vi "对称性1.vi"(11 "XY图":cluster{dbl[], dbl[]}[](graph)) -> (3 "对称性":dbl)   [LabVIEW 2019]
uses:
  <vilib>/Analysis/NI_AAL_Geometry.lvlib
panel:
  out "右":dbl
  out "左":dbl
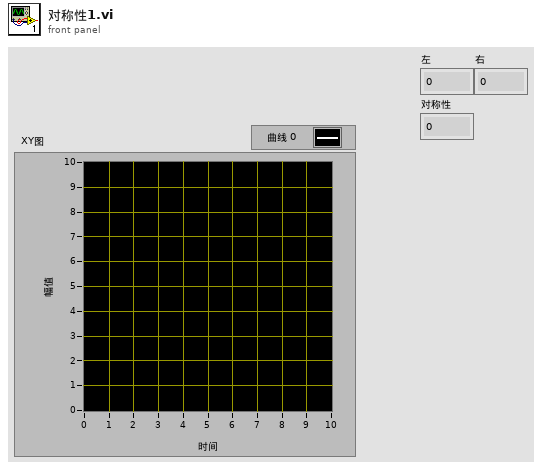
[diagram p1: front panel]
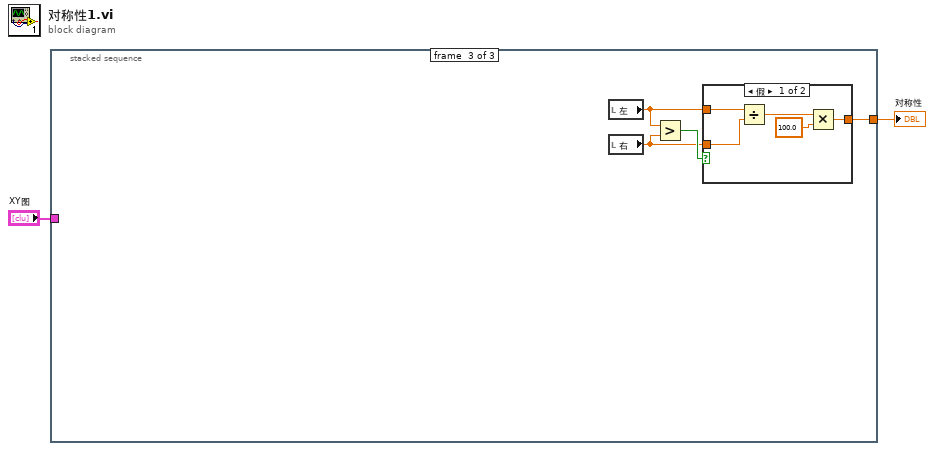
[diagram p0: block diagram]
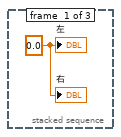
[diagram p2: hidden frame]
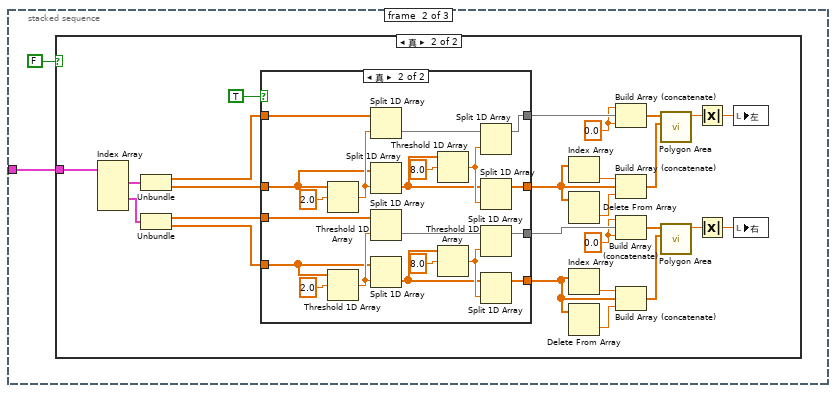
[diagram p3: hidden frame]
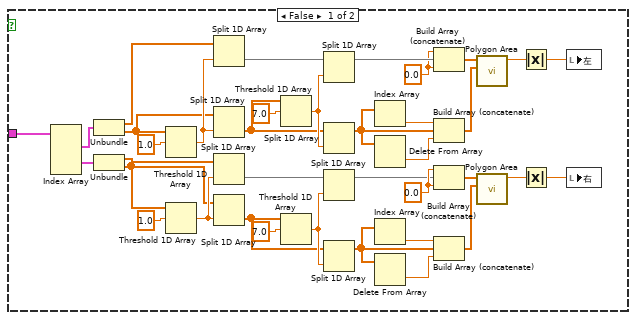
[diagram p4: hidden frame]
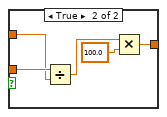
[diagram p6: hidden frame]
diagram:
  n1 = stacked-sequence {
    tunnel: "XY图" -> [_ w4 _]
    tunnel: [_ _ w93] -> w2
    frame #0 {
      w3 = 0.0 ("左")
      "左" <- w3
      "右" <- w3
    }
    frame #1 {
      n2 = case shown="真" FALSE {
        tunnel: w4 -> [w36 w44]
        frame False {
          w10 = 0.0
          w18 = 0.0
          n3 = Index Array(array=w36) -> (element #1=w37:cluster{dbl[], dbl[]}, element #3=w38:cluster{dbl[], dbl[]})  [unwired: 4 in, 2 out]
          n4 = Unbundle(w37) -> (w34:dbl[], w28:dbl[])
          n5 = Unbundle(w38) -> (w29:dbl[], w30:dbl[])
          n6 = Threshold 1D Array(2:1.0 ("阈值y"), 3:w28) -> (0:w33:dbl)  [unwired: 1 in]
          n7 = Threshold 1D Array(2:1.0 ("阈值y"), 3:w30) -> (0:w32:dbl)  [unwired: 1 in]
          n8 = Split 1D Array(array=w34, index=w33) -> (second subarray=w25:dbl[])  [unwired: 1 out]
          n9 = Split 1D Array(array=w28, index=w33) -> (second subarray=w24:dbl[])  [unwired: 1 out]
          n10 = Split 1D Array(array=w29, index=w32) -> (second subarray=w21:dbl[])  [unwired: 1 out]
          n11 = Split 1D Array(array=w30, index=w32) -> (second subarray=w20:dbl[])  [unwired: 1 out]
          n12 = Threshold 1D Array(2:7.0 ("阈值y"), 3:w24) -> (0:w27:dbl)  [unwired: 1 in]
          n13 = Threshold 1D Array(2:7.0 ("阈值y"), 3:w20) -> (0:w22:dbl)  [unwired: 1 in]
          n14 = Split 1D Array(array=w25, index=w27) -> (first subarray=w19:dbl[])  [unwired: 1 out]
          n15 = Split 1D Array(array=w24, index=w27) -> (first subarray=w16:dbl[])  [unwired: 1 out]
          n16 = Split 1D Array(array=w21, index=w22) -> (first subarray=w8:dbl[])  [unwired: 1 out]
          n17 = Split 1D Array(array=w20, index=w22) -> (first subarray=w9:dbl[])  [unwired: 1 out]
          n18 = Index Array(array=w16) -> (element=w17:dbl)  [unwired: 1 in]
          n19 = Delete From Array(array=w16) -> (deleted portion=w15:dbl)  [unwired: 2 in, 1 out]
          n20 = Index Array(array=w9) -> (element=w11:dbl)  [unwired: 1 in]
          n21 = Delete From Array(array=w9) -> (deleted portion=w12:dbl)  [unwired: 2 in, 1 out]
          n22 = Build Array (concatenate)(w18, w19, w18) -> (w14:dbl[])
          n23 = Build Array (concatenate)(w17, w16, w15) -> (w13:dbl[])
          n24 = Build Array (concatenate)(w10, w8, w10) -> (w7:dbl[])
          n25 = Build Array (concatenate)(w11, w9, w12) -> (w6:dbl[])
          n26 = call <vilib>:"Polygon Area.vi"("Y"=w13, "X"=w14) -> ("signed area"=w39:dbl)  [unwired: 8 in, 1 out]
          n27 = call <vilib>:"Polygon Area.vi"("Y"=w6, "X"=w7) -> ("signed area"=w41:dbl)  [unwired: 8 in, 1 out]
          n28 = Absolute Value(x=w39) -> (abs(x)=w40:dbl)
          n29 = Absolute Value(x=w41) -> (abs(x)=w42:dbl)
          n30 = local write "左"(w40) -> ()
          n31 = local write "右"(w42) -> ()
        }
        frame True {
          w46 = 0.0
          w45 = 0.0
          n32 = Index Array(array=w44) -> (element #1=w63:cluster{dbl[], dbl[]}, element #3=w64:cluster{dbl[], dbl[]})  [unwired: 4 in, 2 out]
          n33 = Unbundle(w63) -> (w62:dbl[], w59:dbl[])
          n34 = Unbundle(w64) -> (w60:dbl[], w61:dbl[])
          n35 = case shown="真" TRUE {
            tunnel: w62 -> [w72 w92]
            tunnel: w61 -> [w69 w89]
            tunnel: w60 -> [w70 w88]
            tunnel: w59 -> [w71 w87]
            tunnel: [w72 w80] -> w58
            tunnel: [w71 w79] -> w56
            tunnel: [w69 w78] -> w50
            tunnel: [w70 w77] -> w49
            frame False {
            }
            frame True {
              n36 = Threshold 1D Array(2:2.0 ("阈值y"), 3:w87) -> (0:w91:dbl)  [unwired: 1 in]
              n37 = Threshold 1D Array(2:2.0 ("阈值y"), 3:w89) -> (0:w90:dbl)  [unwired: 1 in]
              n38 = Split 1D Array(array=w92, index=w91) -> (second subarray=w85:dbl[])  [unwired: 1 out]
              n39 = Split 1D Array(array=w87, index=w91) -> (second subarray=w84:dbl[])  [unwired: 1 out]
              n40 = Split 1D Array(array=w88, index=w90) -> (second subarray=w82:dbl[])  [unwired: 1 out]
              n41 = Split 1D Array(array=w89, index=w90) -> (second subarray=w81:dbl[])  [unwired: 1 out]
              n42 = Threshold 1D Array(2:8.0 ("阈值y"), 3:w84) -> (0:w86:dbl)  [unwired: 1 in]
              n43 = Threshold 1D Array(2:8.0 ("阈值y"), 3:w81) -> (0:w83:dbl)  [unwired: 1 in]
              n44 = Split 1D Array(array=w85, index=w86) -> (first subarray=w80:dbl[])  [unwired: 1 out]
              n45 = Split 1D Array(array=w84, index=w86) -> (first subarray=w79:dbl[])  [unwired: 1 out]
              n46 = Split 1D Array(array=w82, index=w83) -> (first subarray=w77:dbl[])  [unwired: 1 out]
              n47 = Split 1D Array(array=w81, index=w83) -> (first subarray=w78:dbl[])  [unwired: 1 out]
            }
          }
          n48 = Index Array(array=w56) -> (element=w57:dbl)  [unwired: 1 in]
          n49 = Delete From Array(array=w56) -> (deleted portion=w55:dbl)  [unwired: 2 in, 1 out]
          n50 = Index Array(array=w50) -> (element=w51:dbl)  [unwired: 1 in]
          n51 = Delete From Array(array=w50) -> (deleted portion=w52:dbl)  [unwired: 2 in, 1 out]
          n52 = Build Array (concatenate)(w45, w58, w45) -> (w54:dbl[])
          n53 = Build Array (concatenate)(w57, w56, w55) -> (w53:dbl[])
          n54 = Build Array (concatenate)(w46, w49, w46) -> (w48:dbl[])
          n55 = Build Array (concatenate)(w51, w50, w52) -> (w47:dbl[])
          n56 = call <vilib>:"Polygon Area.vi"("Y"=w53, "X"=w54) -> ("signed area"=w65:dbl)  [unwired: 8 in, 1 out]
          n57 = call <vilib>:"Polygon Area.vi"("Y"=w47, "X"=w48) -> ("signed area"=w67:dbl)  [unwired: 8 in, 1 out]
          n58 = Absolute Value(x=w65) -> (abs(x)=w66:dbl)
          n59 = Absolute Value(x=w67) -> (abs(x)=w68:dbl)
          n60 = local write "左"(w66) -> ()
          n61 = local write "右"(w68) -> ()
        }
      }
    }
    frame #2 {
      n62 = local read "左"() -> (w94:dbl)
      n63 = local read "右"() -> (w95:dbl)
      n64 = Greater?(x=w94, y=w95) -> (0:w96:bool)
      n65 = case shown="假" w96 {
        tunnel: w95 -> [w100 w106]
        tunnel: w94 -> [w101 w105]
        tunnel: [w97 w103] -> w93
        frame False {
          n66 = Divide(x=w101, y=w100) -> (x/y=w99:dbl)
          n67 = Multiply(x=w99, y=100.0) -> (x*y=w97:dbl)
        }
        frame True {
          n68 = Divide(x=w106, y=w105) -> (x/y=w104:dbl)
          n69 = Multiply(x=w104, y=100.0) -> (x*y=w103:dbl)
        }
      }
    }
  }
  "对称性" <- w2
